vi "Min-SP-GetChannelRefs.vi"(8 "Error In":errorcluster, 9 "OK Button":bool, 11 "Device Ref in":T1 format="%.0x") -> (0 "Error Out":errorcluster, 2 "Group Data Array":T2(array[cluster]) {"VS Refs" format="%.0x"}, 3 "Device Ref out":T1=18446744073709551615 format="%.0x")   [LabVIEW 2017, in "Waveform-Processing-Custom-Device Shared.lvlib" / "Min_SP.lvlib"]
uses:
  Min_SP.lvlib
  <vilib>/NI Veristand/Custom Device API/Custom Device Item Ref.ctl
  Constants.vi
  <vilib>/NI Veristand/Custom Device API/Get Item Property (Dependent Node Pointer).vi
  <vilib>/NI Veristand/Custom Device API/Custom Device API.lvlib
  System Explorer/Waveform-Processing-Custom-Device System Explorer.lvlib
  Waveform-Processing-Custom-Device Shared.lvlib
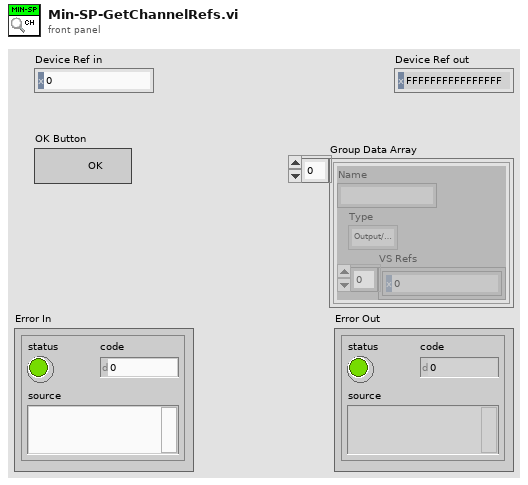
[diagram p1: front panel]
types:
  T1 = typedef "Custom Device API.lvlib/Custom Device Item Ref.ctl" = u64
  T2 = cluster{"Name":string, "Type":enum16{"Output/Write", "Input/Read", "Input/ReadWrite"}, "VS Refs":T1[]}[]
  T3 = enum16{"Output/Write", "Input/Read", "Input/ReadWrite"}
  T4 = cluster{"Name":string, "Type":enum16{"Output/Write", "Input/Read", "Input/ReadWrite"}, "VS Refs":T1[]}
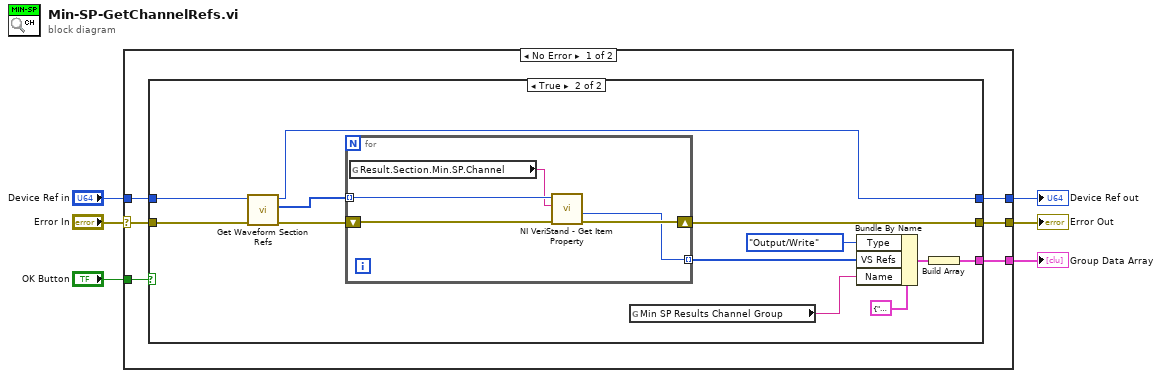
[diagram p0: block diagram]
diagram:
  n1 = case shown="No Error" "Error In" {
    selector: "Error In" -> [w12 w33]
    tunnel: [w10 w33] -> w5
    tunnel: "Device Ref in" -> [w11 w32]
    tunnel: "OK Button" -> [w9 _]
    tunnel: [w8 w32] -> w4
    tunnel: [w7 _] -> w6
    frame No Error {
      n2 = case shown="True" w9 {
        tunnel: w12 -> [w14 w26]
        tunnel: w11 -> [w13 w25]
        tunnel: [w14 w22] -> w10
        tunnel: [w13 w15] -> w8
        tunnel: [_ w16] -> w7
        frame False {
        }
        frame True {
          n3 = call "Get Waveform Section Refs.vi"("Error in"=w26, "Device Ref in"=w25) -> ("Error out"=w24:errorcluster, "Result Section Refs"=w23:T1[], "Device Ref out"=w15:T1)  [unwired: 7 in]
          n4 = for {
            tunnel: w23 -> [w30] mode=indexing
            shift-right: [w29] -> w22
            shift-left: w24 -> [w31]
            tunnel: [w28] -> w21 mode=indexing
            n5 = global read "Constants.vi" "Result.Section.Min.SP.Channel"() -> (w27:string)
            n6 = call-poly <vilib>:"NI VeriStand - Get Item Property.vi"("error in (no error)"=w31, "Property Name"=w27, "Item Ref in"=w30) -> ("error out"=w29:errorcluster, "Dependent Node Ref"=w28:T1)  [unwired: 5 in, 2 out]
          }
          n7 = global read "Constants.vi" "Min SP Results Channel Group"() -> (w18:string)
          n8 = Bundle By Name(cluster=T4 {"Name"="", "Type"=enum."Output/Write", "VS Refs"=[]} ("Group"), "Type"=T3."Output/Write", "VS Refs"=w21, "Name"=w18) -> (w17:T4)
          n9 = Build Array(w17) -> (w16:T2)
        }
      }
    }
    frame Error {
    }
  }
  "Device Ref out" <- w4
  "Group Data Array" <- w6
  "Error Out" <- w5
